vi "Acquire Waveform.vi"(8 "error in (no error)":errorcluster, 10 "Channel Name":string, 11 "Test Scope in":refnum<class "Test Scope.lvclass">) -> (0 "error out":errorcluster, 2 "Waveform":waveform(dbl), 3 "Test Scope out":refnum<class "Test Scope.lvclass">)   [LabVIEW 2015, in "Test Scope.lvclass"]
uses:
  Test Scope.lvclass
  src/Scope/Scope.lvclass
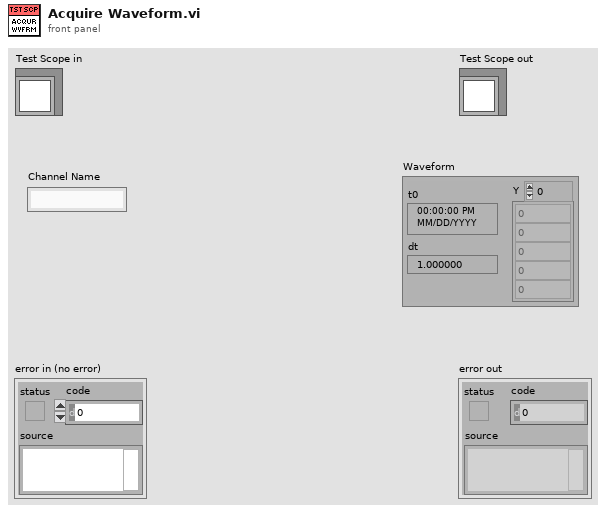
[diagram p1: front panel]
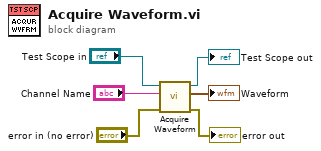
[diagram p0: block diagram]
diagram:
  n1 = call-parent "Acquire Waveform.vi"("error in (no error)"="error in (no error)", "Channel Name"="Channel Name", "Scope in"="Test Scope in") -> ("error out"=→"error out":errorcluster, "Waveform"=→"Waveform":waveform(dbl), "Scope out"=→"Test Scope out":refnum<class "Test Scope.lvclass">)  [unwired: 6 in]
